vi "GUI main.vi"() -> ()   [LabVIEW 2020]
doc: "Use this template to build a producer/consumer design pattern with events to produce queue items. Use this design pattern instead of the User Interface Event Hanadler pattern for user interfaces when you want to execute code asynchronously in response to an event without slowing the user interface responsiveness."
uses:
  Type definitions/FFmeter settings.ctl
  General AC source/Type definitions/AC Source.ctl
  General AC source/Type definitions/AC Source type.ctl
  General DC meter/Type definitions/DC meter.ctl
  General DC meter/Type definitions/DC meter type.ctl
  Measurement/Type definitions/Measuement properties.ctl
  <vilib>/Utility/error.llb/Error Cluster From Error Code.vi
  <vilib>/ErrorRing/Error Ring.xnode
  external libraries/varilib/varilib.lvlib
panel:
  in  "Setup DCV meter":bool
  out "FFmeter settings":T1={"AC Source"={"AC Source type"=enum."Fluke 5XXX calibrator", "VISA"="", "Ref. clock (Hz)"=0.0}, "TWM pipe"="\\\\.\\pipe\\TWM:server", "Measurement status ref"=refnum, "TWM Status ref"=refnum, "Abort ref"=refnum, "AC Source  status ref"=refnum, "DC meter"={"DC meter type"=enum."H/A/K 3458", "DC meter VISA"="", "NPLC"=10, "No of readings"=3}, "Measurement properties"={"Measurement frequencies (Hz)"=[1000.0], "Sampling frequency (Hz)"=500000.0, "Signal amplitude (V)"=4.5, "AC-DC settle time (s)"=20.0, "Record length (multiples of period)"=[1000.0, 10000.0, 1000.0], "Measurement template file"=path "", "Row of START keyword"=1, "Row of STOP keyword"=0}} {"Measurement properties"."Record length (multiples of period)" format="%#_3p"; "Measurement properties"."Sampling frequency (Hz)" format="%#_3p"; "Measurement properties"."Measurement frequencies (Hz)" format="%#_3p"}
  out "Measurement status":string
  in  "Setup AC Source":bool
  in  "Measure":bool
  out "gui_unlock_for_measure":refnum<vi>[](array[refnum])
  out "gui_to_lock":refnum<vi>[](array[refnum])
  in  "Setup meas":bool
  in  "Abort":bool
  out "AC Source status":string
  out "TWM Status":string
  in  "Setup TWM":bool
  in  "About":bool
  in  "Setup pjvs":bool
  in  "Quit":bool
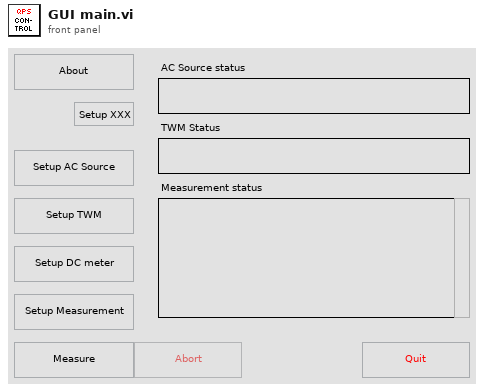
[diagram p1: front panel]
types:
  T1 = typedef "FFmeter settings.ctl" = cluster{"AC Source":T2, "TWM pipe":string, "Measurement status ref":refnum<vi>, "TWM Status ref":refnum<vi>, "Abort ref":refnum<vi>, "AC Source  status ref":refnum<vi>, "DC meter":T4, "Measurement properties":T6}
  T2 = typedef "AC Source.ctl" = cluster{"AC Source type":T3, "VISA":refnum<visa-resource-name>, "Ref. clock (Hz)":dbl}
  T3 = typedef "AC Source type.ctl" = enum16{"Fluke 5XXX calibrator", "Tektronix AFG3101C", "dummy"}
  T4 = typedef "DC meter.ctl" = cluster{"DC meter type":T5, "DC meter VISA":refnum<visa-resource-name>, "NPLC":i32, "No of readings":i32}
  T5 = typedef "DC meter type.ctl" = enum16{"H/A/K 3458", "FLuke 8508A", "dummy"}
  T6 = typedef "Measuement properties.ctl" = cluster{"Measurement frequencies (Hz)":dbl[], "Sampling frequency (Hz)":dbl, "Signal amplitude (V)":dbl, "AC-DC settle time (s)":dbl, "Record length (multiples of period)":dbl[], "Measurement template file":path, "Row of START keyword":i32, "Row of STOP keyword":i32}
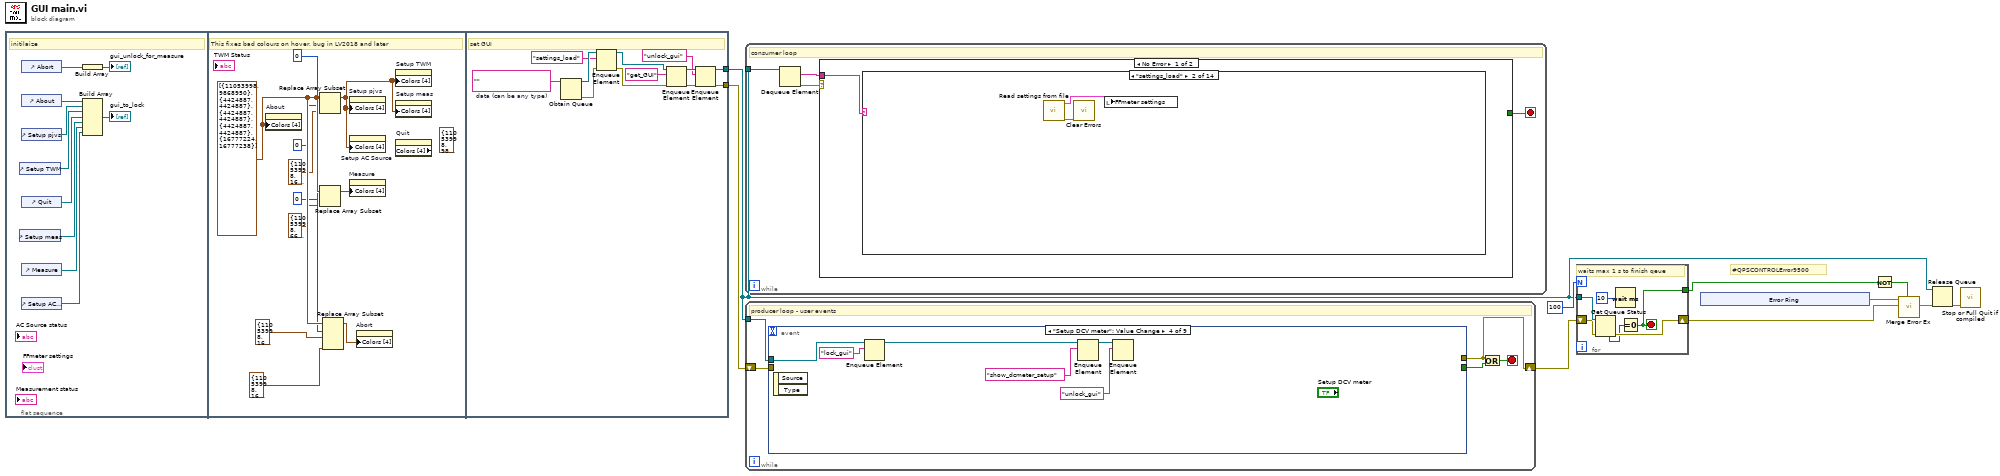
[diagram p0: block diagram]
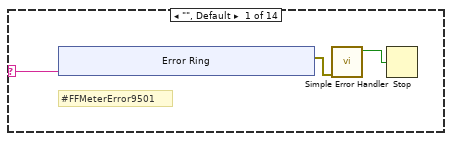
[diagram p2: hidden frame]
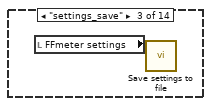
[diagram p3: hidden frame]
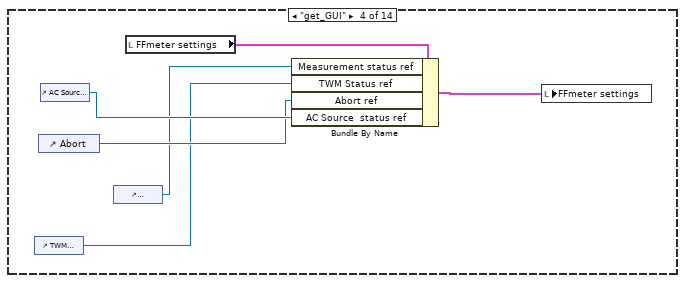
[diagram p4: hidden frame]
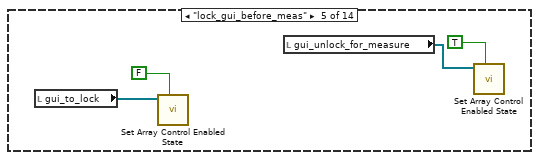
[diagram p5: hidden frame]
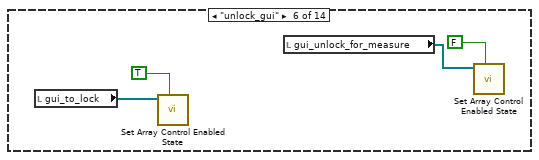
[diagram p6: hidden frame]
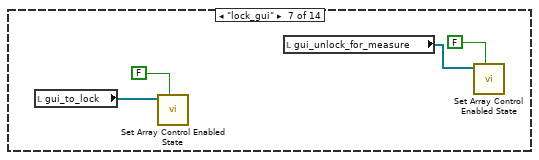
[diagram p7: hidden frame]
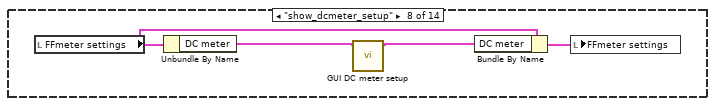
[diagram p8: hidden frame]
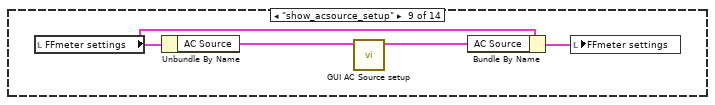
[diagram p9: hidden frame]
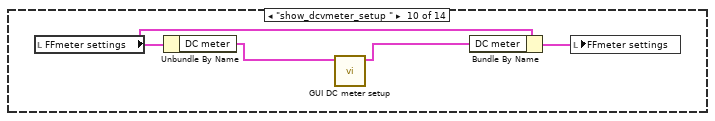
[diagram p10: hidden frame]
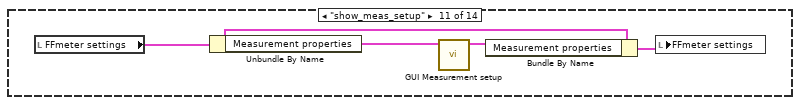
[diagram p11: hidden frame]
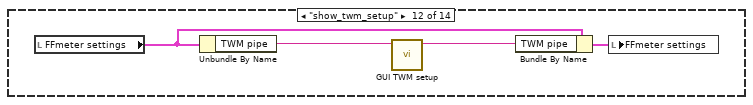
[diagram p12: hidden frame]
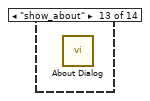
[diagram p13: hidden frame]
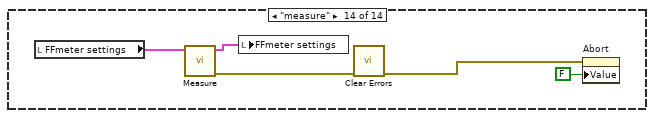
[diagram p14: hidden frame]
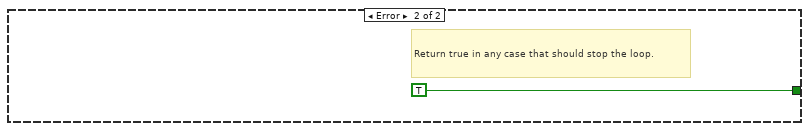
[diagram p15: hidden frame]
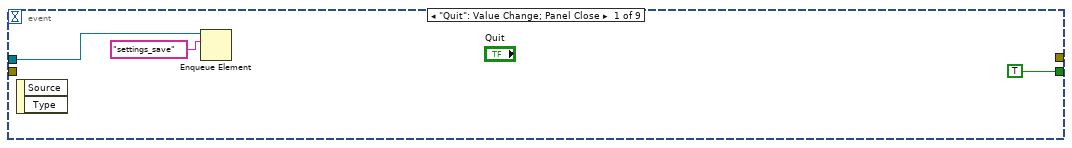
[diagram p16: hidden frame]
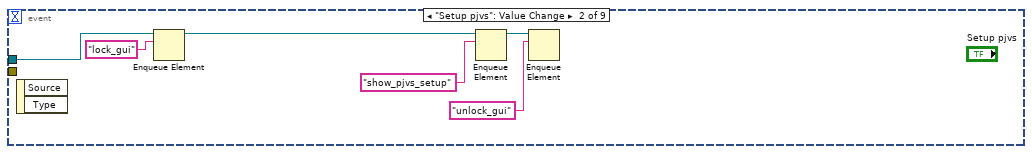
[diagram p17: hidden frame]
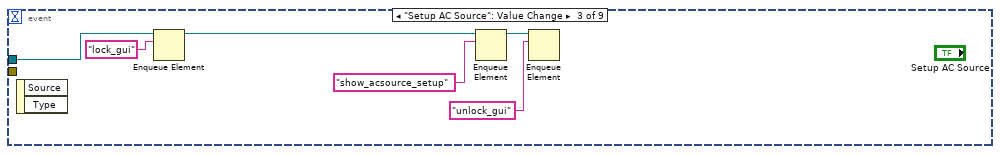
[diagram p18: hidden frame]
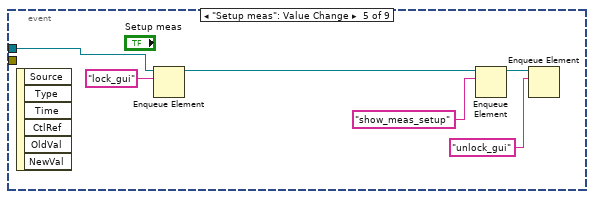
[diagram p19: hidden frame]
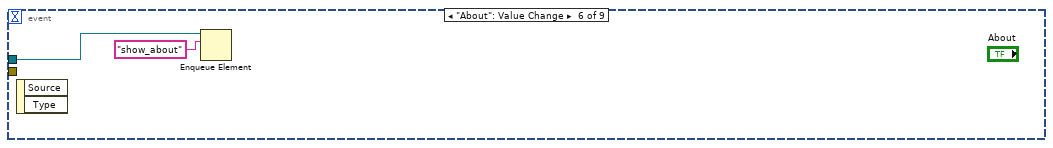
[diagram p20: hidden frame]
diagram:
  # "#QPSCONTROLError9500"
  n1 = flat-sequence {
    tunnel: [w38] -> w4
    tunnel: [w35] -> w10
    frame #0 {
      # "initilaize"
      n2 = control-ref of="Setup TWM"() -> (w15:refnum<vi>)
      n3 = control-ref of="Setup meas"() -> (w17:refnum<vi>)
      n4 = control-ref of="Abort"() -> (w18:refnum<vi>)
      n5 = control-ref of="About"() -> (w13:refnum<vi>)
      n6 = control-ref of="Setup pjvs"() -> (w14:refnum<vi>)
      n7 = control-ref of="Quit"() -> (w16:refnum<vi>)
      n8 = control-ref of="Measure"() -> (w12:refnum<vi>)
      n9 = control-ref of="Setup AC Source"() -> (w11:refnum<vi>)
      n10 = Build Array(w18) -> (→"gui_unlock_for_measure":refnum<vi>[])
      n11 = Build Array(w13, w14, w15, w16, w17, w12, w11) -> (→"gui_to_lock":refnum<vi>[])
    }
    frame #1 {
      (unwired) cluster{u32, u32} {11053998, 9868950}
      w28 = cluster{u32, u32}[] [{11053998, 9868950}, {4424887, 4424887}, {4424887, 4424887}, {4424887, 4424887}, {16777224, 16777238}] ("Colors [4]")
      # "This fixes bad colours on hover, bug in LV2018 and later"
      n12 = property on="About" class="Bool"("Colors [4]"=w28) -> ()  [unwired: 2 in, 2 out]
      n13 = Replace Array Subset(array=w28, new element=cluster{u32, u32} {11053998, 16776960}, index=0) -> (w31:cluster{u32, u32}[])
      n14 = Replace Array Subset(array=w28, new element=cluster{u32, u32} {11053998, 6618880}, index=0) -> (w29:cluster{u32, u32}[])
      n15 = Replace Array Subset(array=w28, new element #1=cluster{u32, u32} {11053998, 16748945}, index #1=0 ("index"), new element #2=cluster{u32, u32} {11053998, 16748945}) -> (w30:cluster{u32, u32}[])  [unwired: 1 in]
      n16 = property on="Setup pjvs" class="Bool"("Colors [4]"=w31) -> ()  [unwired: 2 in, 2 out]
      n17 = property on="Setup AC Source" class="Bool"("Colors [4]"=w31) -> ()  [unwired: 2 in, 2 out]
      n18 = property on="Measure" class="Bool"("Colors [4]"=w29) -> ()  [unwired: 2 in, 2 out]
      n19 = property on="Abort" class="Bool (strict)"("Colors [4]"=w30) -> ()  [unwired: 2 in, 2 out]
      n20 = property on="Setup TWM" class="Bool"("Colors [4]"=w31) -> ()  [unwired: 2 in, 2 out]
      n21 = property on="Setup meas" class="Bool"("Colors [4]"=w31) -> ()  [unwired: 2 in, 2 out]
      n22 = property on="Quit" class="Bool" props=["Colors [4]"]() -> ()  [unwired: 2 in, 3 out]
    }
    frame #2 {
      w43 = ""  # data (can be any type)
      # "set GUI"
      n23 = Obtain Queue(element data type=w43) -> (queue out=w42:refnum<queue>, error out=w41:errorcluster)  [unwired: 4 in, 1 out]
      n24 = Enqueue Element(queue=w42, element="settings_load", error in (no error)=w41) -> (queue out=w33:refnum<queue>, error out=w32:errorcluster)  [unwired: 1 in, 1 out]
      n25 = Enqueue Element(queue=w33, element="get_GUI", error in (no error)=w32) -> (queue out=w36:refnum<queue>, error out=w37:errorcluster)  [unwired: 1 in, 1 out]
      n26 = Enqueue Element(queue=w36, element="unlock_gui", error in (no error)=w37) -> (queue out=w38:refnum<queue>, error out=w35:errorcluster)  [unwired: 1 in, 1 out]
    }
  }
  n27 = while {
    tunnel: w4 -> [w47]
    stop <- w44 stop-if-true
    # "consumer loop"
    n28 = Dequeue Element(queue=w47) -> (element=w45:string, error out=w46:errorcluster)  [unwired: 2 in, 2 out]
    n29 = case shown="No Error" w46 {
      tunnel: w45 -> [w48 _]
      tunnel: [_ TRUE] -> w44
      frame No Error {
        n30 = case shown="\"settings_load\"" w48 {
          selector: w48 -> [w49 _ _ _ _ _ _ _ _ _ _ _ _ _]
          frame "", Default {
            # "#FFMeterError9501"
            n31 = xnode "Error Ring"("parameter 0"=w49) -> ("error out"=w51:errorcluster)
            n32 = call <vilib>:"Simple Error Handler.vi"("error in (no error)"=w51) -> ("error?"=w50:bool)  [unwired: 4 in, 4 out]
            n33 = Stop(stop? (T)=w50) -> ()
          }
          frame "settings_load" {
            n34 = call "Read settings from file.vi"() -> ("error out"=w59:errorcluster, "FFmeter settings"=w60:T1)  [unwired: 10 in]
            n35 = call <vilib>:"Clear Errors.vi"("error in (no error)"=w59) -> ()  [unwired: 5 in, 2 out]
            n36 = local write "FFmeter settings"(w60) -> ()
          }
          frame "settings_save" {
            n37 = local read "FFmeter settings"() -> (w61:T1)
            n38 = call "Save settings to file.vi"("FFmeter settings"=w61) -> ()  [unwired: 10 in, 1 out]
          }
          frame "get_GUI" {
            n39 = control-ref of="TWM Status"() -> (w62:refnum<vi>)
            n40 = control-ref of="Abort"() -> (w64:refnum<vi>)
            n41 = control-ref of="AC Source status"() -> (w65:refnum<vi>)
            n42 = control-ref of="Measurement status"() -> (w63:refnum<vi>)
            n43 = local read "FFmeter settings"() -> (w67:T1)
            n44 = Bundle By Name(cluster=w67, "Measurement status ref"=w63, "TWM Status ref"=w62, "Abort ref"=w64, "AC Source  status ref"=w65) -> (w66:T1)
            n45 = local write "FFmeter settings"(w66) -> ()
          }
          frame "lock_gui_before_meas" {
            n46 = local read "gui_to_lock"() -> (w71:refnum<vi>[])
            n47 = call "Set Array Control Enabled State.vi"("enabled (T)"=FALSE, "reference array in"=w71) -> ()  [unwired: 8 in, 2 out]
            n48 = local read "gui_unlock_for_measure"() -> (w69:refnum<vi>[])
            n49 = call "Set Array Control Enabled State.vi"("enabled (T)"=TRUE, "reference array in"=w69) -> ()  [unwired: 8 in, 2 out]
          }
          frame "unlock_gui" {
            n50 = local read "gui_to_lock"() -> (w75:refnum<vi>[])
            n51 = call "Set Array Control Enabled State.vi"("enabled (T)"=TRUE, "reference array in"=w75) -> ()  [unwired: 8 in, 2 out]
            n52 = local read "gui_unlock_for_measure"() -> (w74:refnum<vi>[])
            n53 = call "Set Array Control Enabled State.vi"("enabled (T)"=FALSE, "reference array in"=w74) -> ()  [unwired: 8 in, 2 out]
          }
          frame "lock_gui" {
            n54 = local read "gui_to_lock"() -> (w79:refnum<vi>[])
            n55 = call "Set Array Control Enabled State.vi"("enabled (T)"=FALSE, "reference array in"=w79) -> ()  [unwired: 8 in, 2 out]
            n56 = local read "gui_unlock_for_measure"() -> (w78:refnum<vi>[])
            n57 = call "Set Array Control Enabled State.vi"("enabled (T)"=FALSE, "reference array in"=w78) -> ()  [unwired: 8 in, 2 out]
          }
          frame "show_dcmeter_setup" {
            n58 = local read "FFmeter settings"() -> (w83:T1)
            n59 = Unbundle By Name(w83) -> ("DC meter"=w81:T4)
            n60 = call "GUI DC meter setup.vi"("DC meter"=w81) -> ("DC meter out"=w80:T4)  [unwired: 10 in]
            n61 = Bundle By Name(cluster=w83, "DC meter"=w80) -> (w82:T1)
            n62 = local write "FFmeter settings"(w82) -> ()
          }
          frame "show_acsource_setup" {
            n63 = local read "FFmeter settings"() -> (w87:T1)
            n64 = Unbundle By Name(w87) -> ("AC Source"=w85:T2)
            n65 = call "GUI AC Source setup.vi"("AC Source"=w85) -> ("AC Source out"=w84:T2)  [unwired: 10 in]
            n66 = Bundle By Name(cluster=w87, "AC Source"=w84) -> (w86:T1)
            n67 = local write "FFmeter settings"(w86) -> ()
          }
          frame "show_dcvmeter_setup " {
            n68 = local read "FFmeter settings"() -> (w91:T1)
            n69 = Unbundle By Name(w91) -> ("DC meter"=w89:T4)
            n70 = call "GUI DC meter setup.vi"("DC meter"=w89) -> ("DC meter out"=w88:T4)  [unwired: 10 in]
            n71 = Bundle By Name(cluster=w91, "DC meter"=w88) -> (w90:T1)
            n72 = local write "FFmeter settings"(w90) -> ()
          }
          frame "show_meas_setup" {
            n73 = local read "FFmeter settings"() -> (w95:T1)
            n74 = Unbundle By Name(w95) -> ("Measurement properties"=w93:T6)
            n75 = call "GUI Measurement setup.vi"("Measurement properties"=w93) -> ("Measurement properties out"=w92:T6)  [unwired: 10 in]
            n76 = Bundle By Name(cluster=w95, "Measurement properties"=w92) -> (w94:T1)
            n77 = local write "FFmeter settings"(w94) -> ()
          }
          frame "show_twm_setup" {
            n78 = local read "FFmeter settings"() -> (w99:T1)
            n79 = Unbundle By Name(w99) -> ("TWM pipe"=w97:string)
            n80 = call "GUI TWM setup.vi"("TWM pipe"=w97) -> ("TWM pipe out"=w96:string)  [unwired: 10 in]
            n81 = Bundle By Name(cluster=w99, "TWM pipe"=w96) -> (w98:T1)
            n82 = local write "FFmeter settings"(w98) -> ()
          }
          frame "show_about" {
            n83 = call "About Dialog.vi"() -> ()  [unwired: 12 in]
          }
          frame "measure" {
            n84 = local read "FFmeter settings"() -> (w104:T1)
            n85 = call "Measure.vi"("FFmeter settings"=w104) -> ("error out"=w103:errorcluster, "FFmeter settings out"=w100:T1)  [unwired: 9 in]
            n86 = local write "FFmeter settings"(w100) -> ()
            n87 = call <vilib>:"Clear Errors.vi"("error in (no error)"=w103) -> ("error out"=w102:errorcluster)  [unwired: 5 in, 1 out]
            n88 = property on="Abort" class="Bool (strict)"(error in=w102, "Value"=FALSE ("Abort")) -> ()  [unwired: 1 in, 2 out]
          }
        }
      }
      frame Error {
        # "Return true in any case that should stop the loop."
      }
    }
  }
  n89 = while {
    shift-right: [w106] -> w3
    shift-left: w10 -> [w109]
    tunnel: w4 -> [w110]
    stop <- w107 stop-if-true
    # "producer loop - user events"
    n90 = event shown="[3] \"Setup DCV meter\": Value Change" {
      selector: _ -> [_ _ _ _ _ _ _ _ _]
      dyn-events: _ -> [_ _ _ _ _ _ _ _ _]
      timeout: _ -> [_ _ _ _ _ _ _ _ _]
      tunnel: w110 -> [w111 w116 w122 w128 w134 w138 w142 w151 _]
      tunnel: w109 -> [_ _ _ _ _ _ _ _ _]
      tunnel: [_ _ _ _ _ _ _ w146 _] -> w106
      tunnel: [TRUE ("cancel") _ _ _ _ _ _ _ _] -> w108
      event "Quit": Value Change; Panel Close {
        n91 = event-data() -> ()  [unwired: 1 in, 2 out]
        n92 = Enqueue Element(queue=w111, element="settings_save") -> ()  [unwired: 2 in, 3 out]
      }
      event "Setup pjvs": Value Change {
        n93 = event-data() -> ()  [unwired: 1 in, 2 out]
        n94 = Enqueue Element(queue=w116, element="lock_gui") -> (queue out=w115:refnum<queue>)  [unwired: 2 in, 2 out]
        n95 = Enqueue Element(queue=w115, element="show_pjvs_setup") -> (queue out=w114:refnum<queue>)  [unwired: 2 in, 2 out]
        n96 = Enqueue Element(queue=w114, element="unlock_gui") -> ()  [unwired: 2 in, 3 out]
      }
      event "Setup AC Source": Value Change {
        n97 = event-data() -> ()  [unwired: 1 in, 2 out]
        n98 = Enqueue Element(queue=w122, element="lock_gui") -> (queue out=w121:refnum<queue>)  [unwired: 2 in, 2 out]
        n99 = Enqueue Element(queue=w121, element="show_acsource_setup") -> (queue out=w120:refnum<queue>)  [unwired: 2 in, 2 out]
        n100 = Enqueue Element(queue=w120, element="unlock_gui") -> ()  [unwired: 2 in, 3 out]
      }
      event "Setup DCV meter": Value Change {
        n101 = event-data() -> ()  [unwired: 1 in, 2 out]
        n102 = Enqueue Element(queue=w128, element="lock_gui") -> (queue out=w127:refnum<queue>)  [unwired: 2 in, 2 out]
        n103 = Enqueue Element(queue=w127, element="show_dcmeter_setup") -> (queue out=w126:refnum<queue>)  [unwired: 2 in, 2 out]
        n104 = Enqueue Element(queue=w126, element="unlock_gui") -> ()  [unwired: 2 in, 3 out]
      }
      event "Setup meas": Value Change {
        n105 = event-data() -> ()  [unwired: 1 in, 6 out]
        n106 = Enqueue Element(queue=w134, element="lock_gui") -> (queue out=w133:refnum<queue>)  [unwired: 2 in, 2 out]
        n107 = Enqueue Element(queue=w133, element="show_meas_setup") -> (queue out=w132:refnum<queue>)  [unwired: 2 in, 2 out]
        n108 = Enqueue Element(queue=w132, element="unlock_gui") -> ()  [unwired: 2 in, 3 out]
      }
      event "About": Value Change {
        n109 = event-data() -> ()  [unwired: 1 in, 2 out]
        n110 = Enqueue Element(queue=w138, element="show_about") -> ()  [unwired: 2 in, 3 out]
      }
      event "Setup TWM": Value Change {
        n111 = event-data() -> ()  [unwired: 1 in, 2 out]
        n112 = Enqueue Element(queue=w142, element="lock_gui") -> (queue out=w141:refnum<queue>)  [unwired: 2 in, 2 out]
        n113 = Enqueue Element(queue=w141, element="show_twm_setup") -> (queue out=w140:refnum<queue>)  [unwired: 2 in, 2 out]
        n114 = Enqueue Element(queue=w140, element="unlock_gui") -> ()  [unwired: 2 in, 3 out]
      }
      event "Measure": Value Change {
        n115 = event-data() -> ()  [unwired: 1 in, 6 out]
        n116 = Enqueue Element(queue=w151, element="lock_gui_before_meas") -> (queue out=w150:refnum<queue>)  [unwired: 2 in, 2 out]
        n117 = Enqueue Element(queue=w150, element="measure") -> (queue out=w149:refnum<queue>)  [unwired: 2 in, 2 out]
        n118 = Enqueue Element(queue=w149, element="unlock_gui") -> (error out=w146:errorcluster)  [unwired: 2 in, 2 out]
      }
      event "Abort": Value Change {
        n119 = event-data() -> ()  [unwired: 1 in, 6 out]
        n120 = control-ref of="Abort"() -> (w154:refnum<vi>)
        n121 = call "Set Control Enabled State.vi"("enabled (T)"=FALSE, "reference in"=w154) -> ()  [unwired: 8 in, 2 out]
      }
    }
    n122 = Or(x=w106, y=w108) -> (x .or. y?=w107:bool)
  }
  n123 = for {
    N: 100 -> [_]
    tunnel: w4 -> [w160]
    shift-right: [w158] -> w8
    shift-left: w3 -> [w159]
    tunnel: [w155] -> w6
    stop <- w155 stop-if-true
    # "waits max 1 s to finish qeue"
    n124 = Get Queue Status(queue=w160, error in (no error)=w159) -> (error out=w158:errorcluster, # elements in queue=w156:i32)  [unwired: 1 in, 6 out]
    n125 = Wait (ms)(milliseconds to wait=u32 10) -> ()  [unwired: 1 out]
    n126 = Equal To 0?(x=w156) -> (x = 0?=w155:bool)
  }
  n127 = xnode "Error Ring"() -> ("error out"=w9:errorcluster)
  n128 = Not(x=w6) -> (.not. x?=w7:bool)
  n129 = call "Merge Error Ex.vi"("Is error? (False)"=w7, "main error in (no error)"=w8, "second error in"=w9) -> ("error out"=w2:errorcluster)  [unwired: 8 in]
  n130 = Release Queue(queue=w4, error in (no error)=w2) -> (error out=w1:errorcluster)  [unwired: 1 in, 2 out]
  n131 = call "Stop or Full Quit if compiled.vi"("error in (no effect)"=w1) -> ()  [unwired: 3 in]
